vi "Add.vi"(4 "case matching (sensitive)":T1=enum."system", 5 "value":string, 6 "key":string, 7 "array in":T2) -> (1 "replaced":bool, 2 "prev value":string, 3 "array out":T2)   [LabVIEW 2009, in "Tools_KeyedArray.lvlib"]
doc: "Adds a new element identified by <B>key</B> and containing <B>value</B> to <B>array in</B>."
uses:
  Tools_KeyedArray.lvlib
  KeyedArray.ctl
  <vilib>/NI/Tools/String/Case Matching.ctl
  <vilib>/NI/Tools/String/Tools_String.lvlib
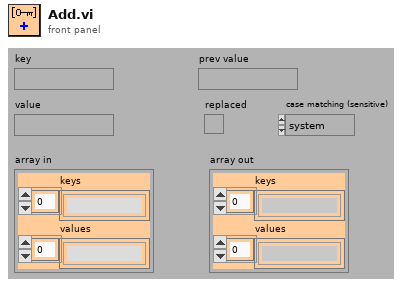
[diagram p1: front panel]
types:
  T1 = typedef "Tools_String.lvlib/Case Matching.ctl" = enum16{"a != A", "a == A", "system"}
  T2 = typedef "Tools_KeyedArray.lvlib/KeyedArray.ctl" = cluster{"keys":string[], "values":string[]}
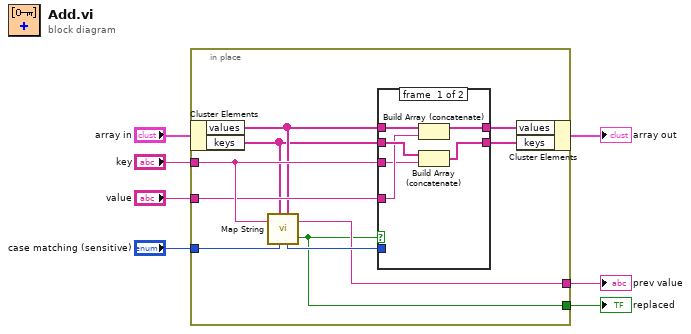
[diagram p0: block diagram]
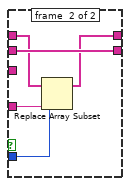
[diagram p2: hidden frame]
diagram:
  n1 = in-place {
    in-place-border: "key" -> [w17]
    in-place-border: "value" -> [w16]
    in-place-border: [w14] -> w5
    in-place-border: [w13] -> w4
    in-place-border: "case matching (sensitive)" -> [w12]
    n2 = in-place-cluster #1("array in") -> ("values"=w11:string[], "keys"=w10:string[])
    n3 = call "Map String.vi"("case matching (sensitive)"=w12, "key"=w17, "keys"=w10, "values"=w11) -> ("index"=w15:i32, "valid key"=w13:bool, "value"=w14:string)  [unwired: 1 in]
    n4 = case shown="True" w13 {
      tunnel: w16 -> [w19 w25]
      tunnel: w17 -> [w18 _]
      tunnel: w10 -> [w23 w28]
      tunnel: w11 -> [w22 w27]
      tunnel: [w21 w28] -> w8
      tunnel: [w20 w26] -> w9
      tunnel: w15 -> [_ w24]
      frame #0 {
        n5 = Build Array (concatenate)(w22, w19) -> (w20:string[])
        n6 = Build Array (concatenate)(w23, w18) -> (w21:string[])
      }
      frame #1 {
        n7 = Replace Array Subset(array=w27, new element=w25, index=w24) -> (w26:string[])
      }
    }
    n8 = in-place-cluster #1("values"=w9, "keys"=w8) -> (→"array out":T2)
  }
  "replaced" <- w4
  "prev value" <- w5
